vi "sender_info_finder.vi"(1 "error (in)":errorcluster, 2 "service name":string, 3 "file (use dialog)":path) -> (0 "error (out)":errorcluster)   [LabVIEW 2016]
doc: "Grab the .project8_authentications.json file in the home and read the AMQP credentials."
uses:
  global/sender_info.vi
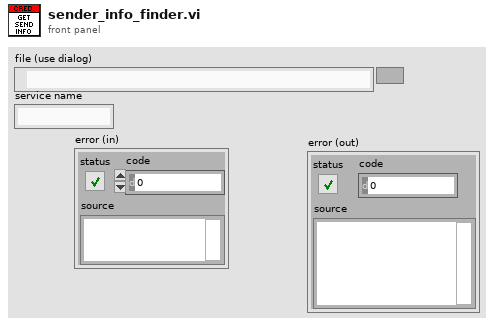
[diagram p1: front panel]
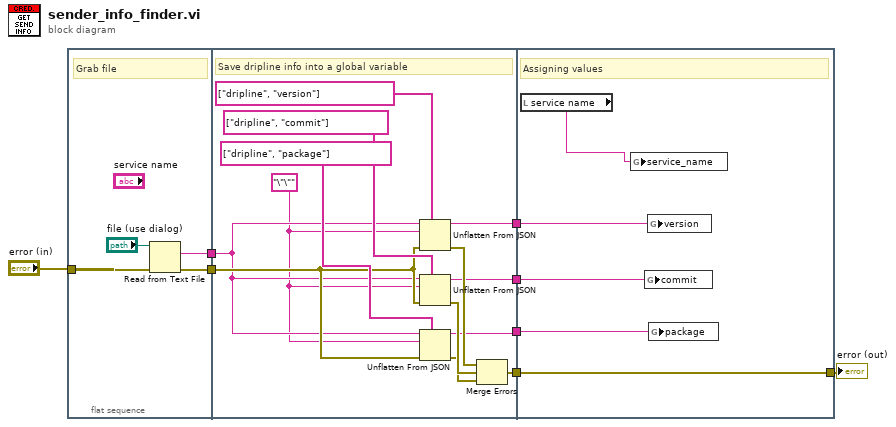
[diagram p0: block diagram]
diagram:
  n1 = flat-sequence {
    tunnel: [w12] -> w8
    tunnel: [w11] -> w7
    tunnel: "error (in)" -> [w10]
    tunnel: w8 -> [w16]
    tunnel: w7 -> [w17]
    tunnel: [w21] -> w4
    tunnel: [w20] -> w3
    tunnel: [w19] -> w2
    tunnel: [w15] -> w1
    tunnel: [w30] -> w6
    tunnel: w4 -> [w30]
    tunnel: w3 -> [w29]
    tunnel: w2 -> [w28]
    tunnel: w1 -> [w27]
    frame #0 {
      # "Grab file"
      n2 = Read from Text File(file (use dialog)="file (use dialog)", error in=w10) -> (text=w12:string, error out=w11:errorcluster)  [unwired: 2 in, 2 out]
    }
    frame #1 {
      w13 = "\"\""
      # "Save dripline info into a global variable"
      n3 = Unflatten From JSON(path=string[] ["dripline", "version"], JSON string=w16, type and defaults=w13, error in (no error)=w17) -> (value=w20:string, error out=w23:errorcluster)  [unwired: 3 in]
      n4 = Unflatten From JSON(path=string[] ["dripline", "commit"], JSON string=w16, type and defaults=w13, error in (no error)=w17) -> (value=w19:string, error out=w22:errorcluster)  [unwired: 3 in]
      n5 = Unflatten From JSON(path=string[] ["dripline", "package"], JSON string=w16, type and defaults=w13, error in (no error)=w17) -> (value=w15:string, error out=w14:errorcluster)  [unwired: 3 in]
      n6 = Merge Errors(w23, w22, w14) -> (w21:errorcluster)
    }
    frame #2 {
      # "Assigning values"
      n7 = local read "service name"() -> (w26:string)
      n8 = global write "sender_info.vi" "service_name"(w26) -> ()
      n9 = global write "sender_info.vi" "commit"(w28) -> ()
      n10 = global write "sender_info.vi" "version"(w29) -> ()
      n11 = global write "sender_info.vi" "package"(w27) -> ()
    }
  }
  "error (out)" <- w6
